vi "STD.vi"(0 "System no.":i32=1 min=1 max=4 step=1, 1 "Table Type":u32=1, 2 "Table ID":u32=1, 3 "Data":string, 5 "error in":errorcluster) -> (19 "error out":errorcluster)   [LabVIEW 2020]
doc: "Saves the content of a given table from volatile memory to a data file in nonvolatile memory.\nWith header tables, STD is also used to write the information in the table before it is saved to data file in nonvolatile memory.\n\nE-754: Check HLP? answer to find out if STD is supported"
panel:
  # "Saves the content of a given table from volatile memory to a data file in nonvolatile memory."
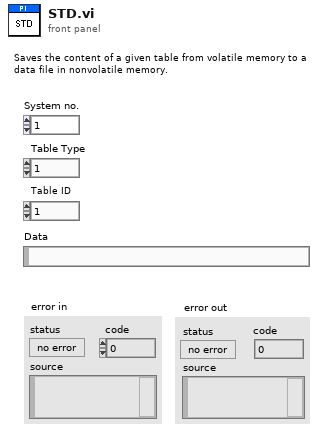
[diagram p1: front panel]
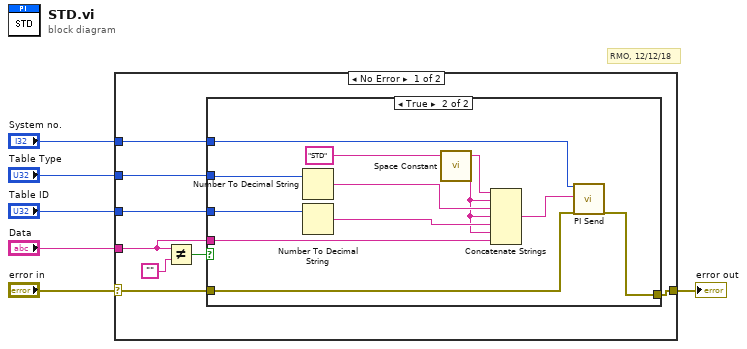
[diagram p0: block diagram]
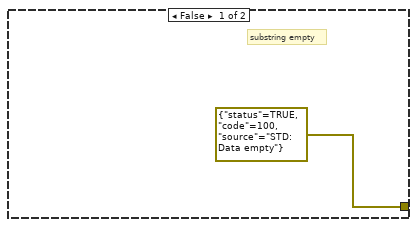
[diagram p2: hidden frame]
diagram:
  # "RMO, 12/12/18"
  n1 = case shown="No Error" "error in" {
    selector: "error in" -> [w13 w27]
    tunnel: [w14 w27] -> w6
    tunnel: "System no." -> [w12 _]
    tunnel: "Data" -> [w7 _]
    tunnel: "Table ID" -> [w8 _]
    tunnel: "Table Type" -> [w9 _]
    frame No Error {
      n2 = Not Equal?(x=w7, y="") -> (x != y?=w10:bool)
      n3 = case shown="True" w10 {
        tunnel: [errorcluster {"status"=TRUE, "code"=100, "source"="STD: Data empty"} ("error out") w25] -> w14
        tunnel: w13 -> [_ w26]
        tunnel: w12 -> [_ w24]
        tunnel: w9 -> [_ w23]
        tunnel: w8 -> [_ w22]
        tunnel: w7 -> [_ w16]
        frame False {
          # "substring empty"
        }
        frame True {
          n4 = Number To Decimal String(number=w23) -> (decimal integer string=w19:string)  [unwired: 1 out]
          n5 = Number To Decimal String(number=w22) -> (decimal integer string=w18:string)  [unwired: 1 out]
          n6 = call "Space Constant.vi"() -> ("String"=w17:string)
          n7 = Concatenate Strings("STD", w17, w19, w17, w18, w17, w16) -> (w21:string)
          n8 = call "PI Send.vi"("System no."=w24, "String to send"=w21, "error in"=w26) -> ("error out"=w25:errorcluster)  [unwired: 3 in, 13 out]
        }
      }
    }
    frame Error {
    }
  }
  "error out" <- w6
